vi "PlotPulses.vi"(8 "error in (no error)":errorcluster, 11 "Numeric":i32) -> (0 "error out":errorcluster, 3 "Waveform Graph 2":dbl[](graph))   [LabVIEW 2021]
panel:
  out "ImpulseSig":dbl[](array[numeric])
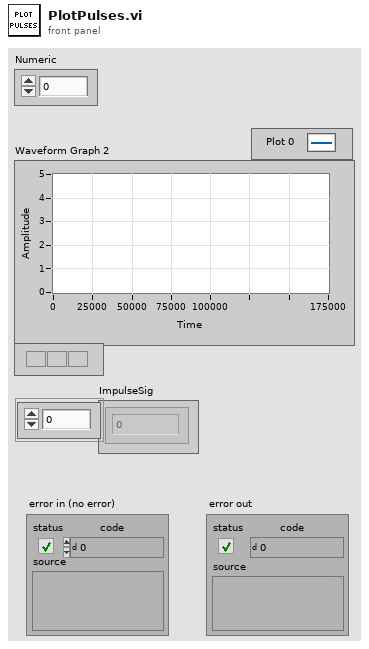
[diagram p1: front panel]
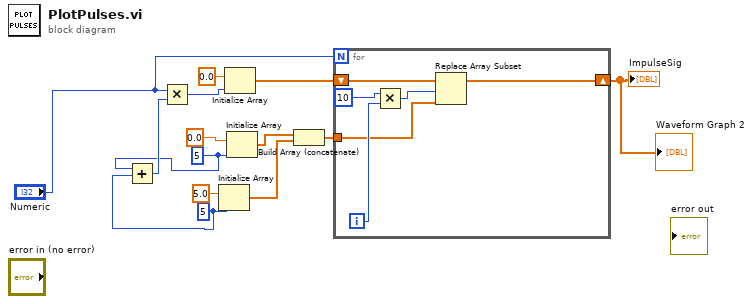
[diagram p0: block diagram]
diagram:
  w7 = 5 ("dimension size")
  w6 = 5 ("dimension size")
  n1 = Add(x=w6, y=w7) -> (x+y=w8:i32)
  n2 = Multiply(x="Numeric", y=w8) -> (x*y=w9:i32)
  n3 = Initialize Array "Initialize Array"(5.0 ("element"), w7) -> (w4:dbl[])
  n4 = Initialize Array "Initialize Array"(0.0 ("element"), w9) -> (w12:dbl[])
  n5 = Initialize Array "Initialize Array"(0.0 ("element"), w6) -> (w3:dbl[])
  n6 = Build Array (concatenate)(w3, w4) -> (w11:dbl[])
  n7 = for {
    N: "Numeric" -> [_]
    tunnel: w11 -> [w16]
    shift-right: [w15] -> w13
    shift-left: w12 -> [w14]
    i -> [w18]
    n8 = Multiply(x=10 ("y"), y=w18) -> (x*y=w17:i32)
    n9 = Replace Array Subset "Replace Array Subset"(array=w14, new element=w16, index=w17) -> (w15:dbl[])
  }
  "ImpulseSig" <- w13
  "Waveform Graph 2" <- w13
